vi "save to xml daq.vi"() -> ()   [LabVIEW 2013, in "DAQ.lvclass"]
uses:
  DAQ.lvclass
  DAQ.lvclass/DAQ.ctl
  <vilib>/Utility/xml.llb/Write to XML File(string).vi
panel:
  in  "?":refnum<class "DAQ.lvclass">
  # "Invoke me to save the class in XML"
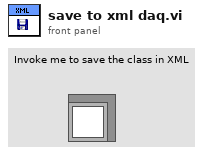
[diagram p1: front panel]
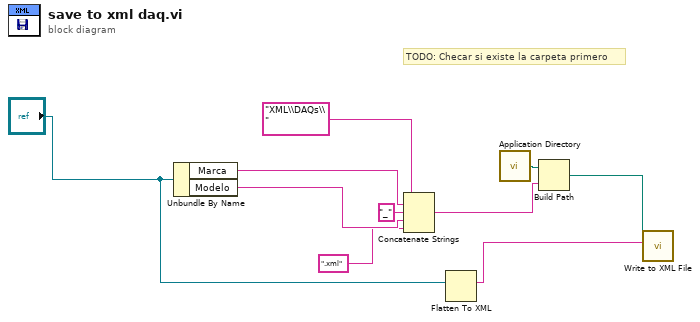
[diagram p0: block diagram]
diagram:
  # "TODO: Checar si existe la carpeta primero"
  n1 = Unbundle By Name("?") -> ("Marca"=w10:string, "Modelo"=w8:string)
  n2 = Concatenate Strings("XML\\DAQs\\" ("string"), w10, "_" ("string"), w8, ".xml" ("string")) -> (w4:string)
  n3 = Flatten To XML(anything="?") -> (xml string=w1:string)
  n4 = call <vilib>:"Application Directory.vi"() -> ("Application Directory"=w5:path)
  n5 = Build Path(base path=w5, name or relative path=w4) -> (appended path=w3:path)
  n6 = call-poly <vilib>:"Write to XML File.vi"("XML Input"=w1, "XML File Path"=w3) -> ()  [unwired: 7 in, 3 out]
